vi "16-2.vi"() -> ()   [LabVIEW 2019, in "16.lvlib"]
uses:
  16.lvlib
panel:
  out "Remaining BITS":bool[](array[boolean])
  out "Result":u64
  out "Version Sum":u32
  out "Packet":T1
  in  "Sample Index":i32
  in  "Sample":bool=TRUE
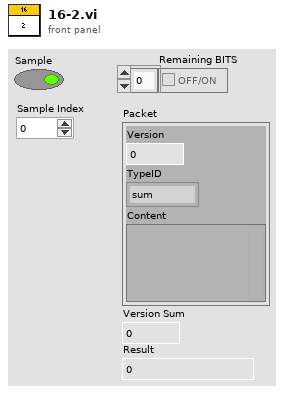
[diagram p1: front panel]
types:
  T1 = cluster{"Version":u32, "TypeID":enum16{"sum", "product", "minimum", "maximum", "literal", "greater than", "less than", "equal to"}, "Content":variant}
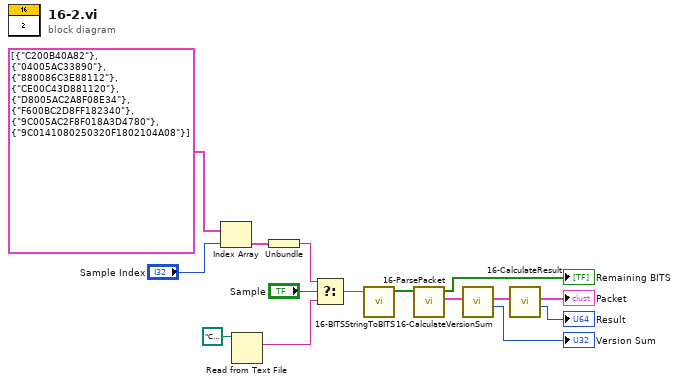
[diagram p0: block diagram]
diagram:
  n1 = Index Array(array=cluster{string}[] [{"C200B40A82"}, {"04005AC33890"}, {"880086C3E88112"}, {"CE00C43D881120"}, {"D8005AC2A8F08E34"}, {"F600BC2D8FF182340"}, {"9C005AC2F8F018A3D4780"}, {"9C0141080250320F1802104A08"}], index="Sample Index") -> (element=w13:cluster{string})
  n2 = Read from Text File(file (use dialog)=path "C:/Users/craig.walker/Documents/GitHub/lv2019-Advent-of-Code-2021/16/input.txt") -> (text=w9:string)  [unwired: 3 in, 3 out]
  n3 = Unbundle(w13) -> (w10:string)
  n4 = Select(t=w10, s="Sample", f=w9) -> (s? t:f=w11:string)
  n5 = call "16-BITSStringToBITS.vi"("BITS String"=w11) -> ("BITS out"=w15:bool[])  [unwired: 10 in]
  n6 = call "16-ParsePacket.vi"("BITS in"=w15) -> ("Packet"=w6:T1, "BITS out"=→"Remaining BITS":bool[])  [unwired: 9 in]
  n7 = call "16-CalculateVersionSum.vi"("Packet in"=w6) -> ("Version Sum"=→"Version Sum":u32, "Packet out"=w4:T1)  [unwired: 9 in]
  n8 = call "16-CalculateResult.vi"("Packet in"=w4) -> ("Result"=→"Result":u64, "Packet out"=→"Packet":T1)  [unwired: 9 in]
